vi "x-axis.vi"(8 "error in (no error)":errorcluster, 11 "Continuous in":refnum<class "Continuous.lvclass">) -> (0 "error out":errorcluster, 1 "Label":string, 2 "Unit":string, 3 "Continuous out":refnum<class "Continuous.lvclass">)   [LabVIEW 2017, in "Continuous.lvclass"]
uses:
  Continuous.lvclass
  Scanner/Scanner.lvclass
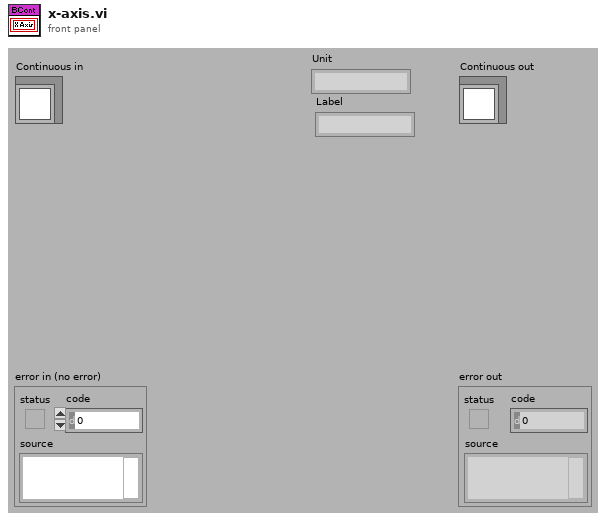
[diagram p1: front panel]
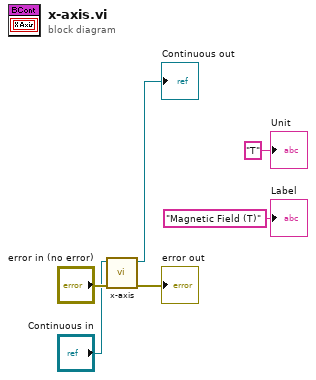
[diagram p0: block diagram]
diagram:
  n1 = call-parent "x-axis.vi"("error in (no error)"="error in (no error)", "Scanner in"="Continuous in") -> ("error out"=→"error out":errorcluster, "Scanner out"=→"Continuous out":refnum<class "Continuous.lvclass">)  [unwired: 6 in, 2 out]
  "Label" <- "Magnetic Field (T)" ("Label")
  "Unit" <- "T" ("Unit")
